vi "Setting.vi"() -> ()   [LabVIEW 2020]
uses:
  <userlib>/_MGI/1D Array/MGI Average/MGI Average (DBL[]).vi
  Libraries/S7/S7.lvlib
panel:
  in  "输出轴大量程标定":bool
  in  "停止":bool
  in  "输出轴小量程标定":bool
  in  "输入轴标定":bool
  out "标定曲线":cluster{dbl[], dbl[]}[](graph)
  # "配置标定"
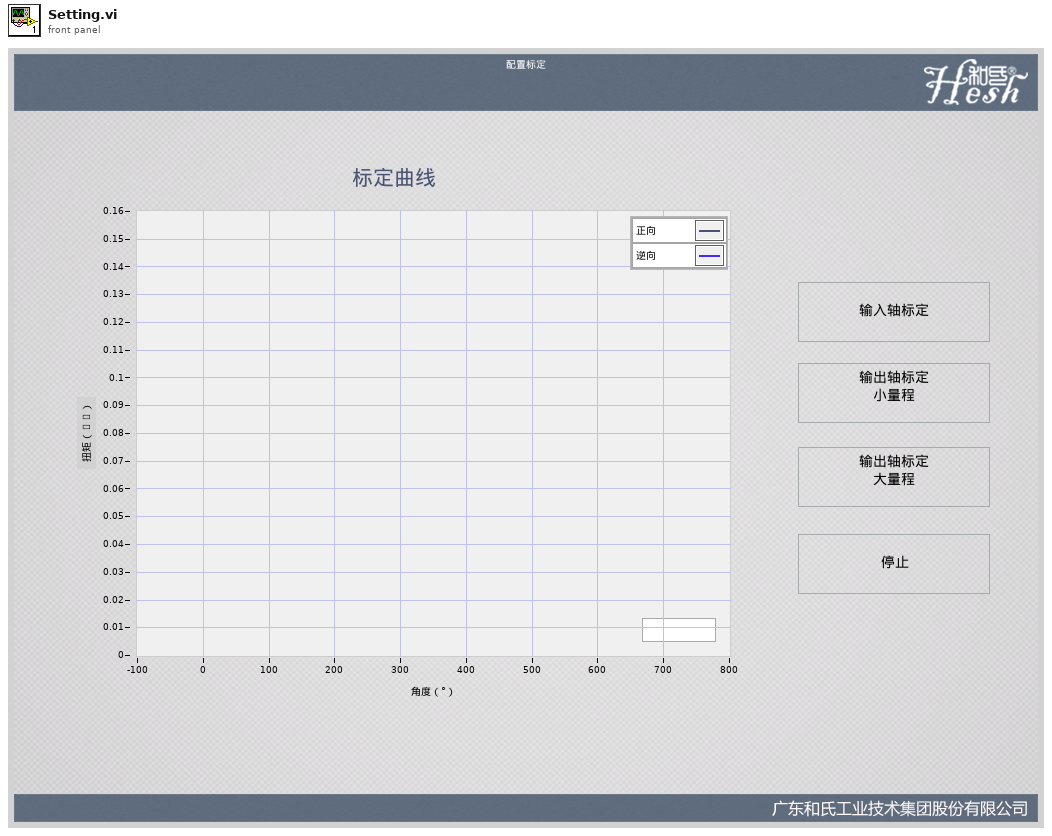
[diagram p1: front panel]
types:
  T1 = cluster{"输入旋转位移":sgl, "输入移载位移":sgl, "工装移载位移":sgl, "输入编码位移":sgl, "输入扭矩":sgl, "输出扭矩(小)":sgl, "输出扭矩(大)":sgl, "吸收电流":sgl, "Factorysensor":sgl, "输出轴旋转角度":sgl, "输出轴移栽位移":sgl, "Factorysensor2":sgl}
  T2 = cluster{"输入轴扭矩":dbl, "输出轴扭矩小量程":dbl, "输出轴扭矩大量程":dbl}
  T3 = typedef "S7.lvlib/Read_Data (Reply Payload)--cluster.ctl" = cluster{"读取成功":bool, "数据":u32[], "Read_Data_error":errorcluster}
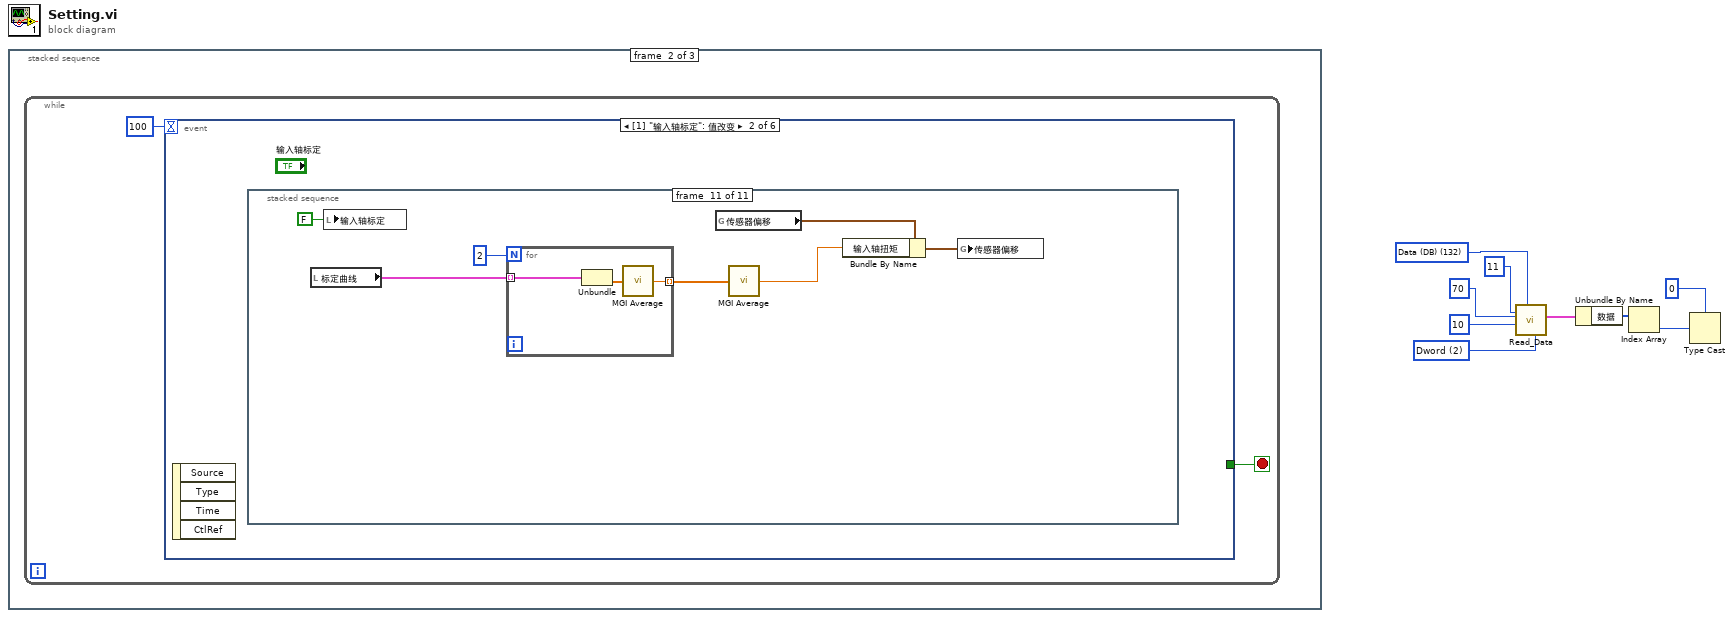
[diagram p0: block diagram]
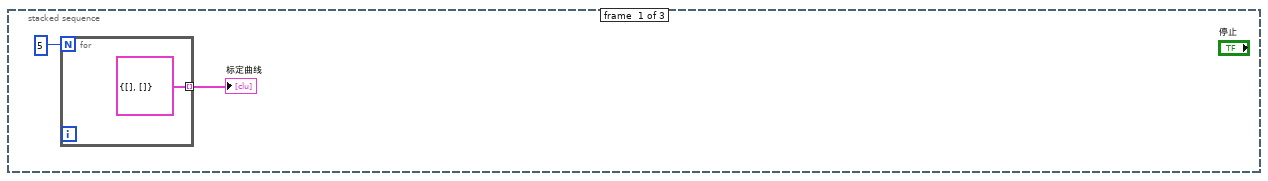
[diagram p2: hidden frame]
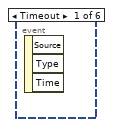
[diagram p3: hidden frame]
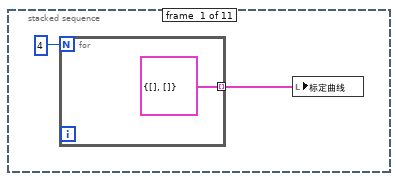
[diagram p4: hidden frame]
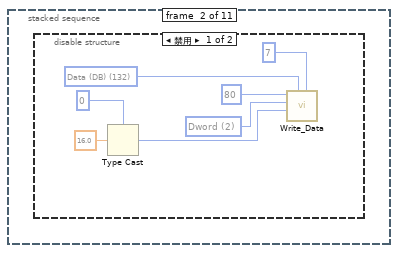
[diagram p5: hidden frame]
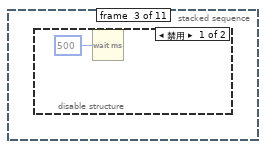
[diagram p7: hidden frame]
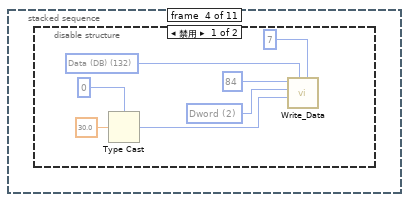
[diagram p9: hidden frame]
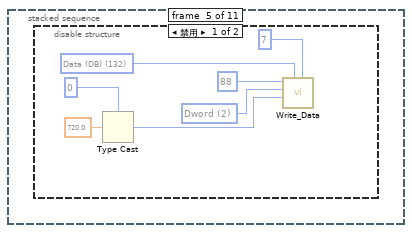
[diagram p11: hidden frame]
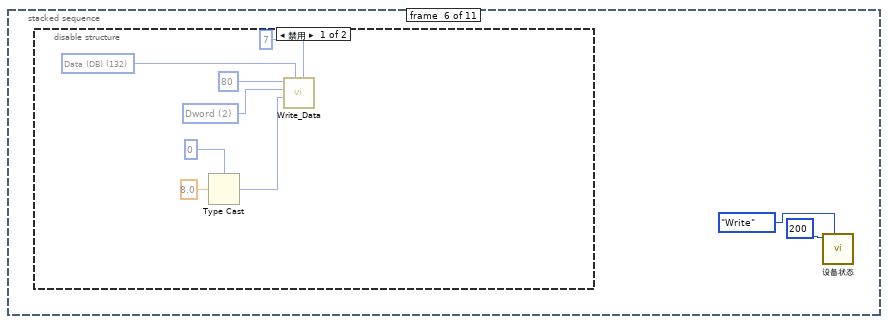
[diagram p13: hidden frame]
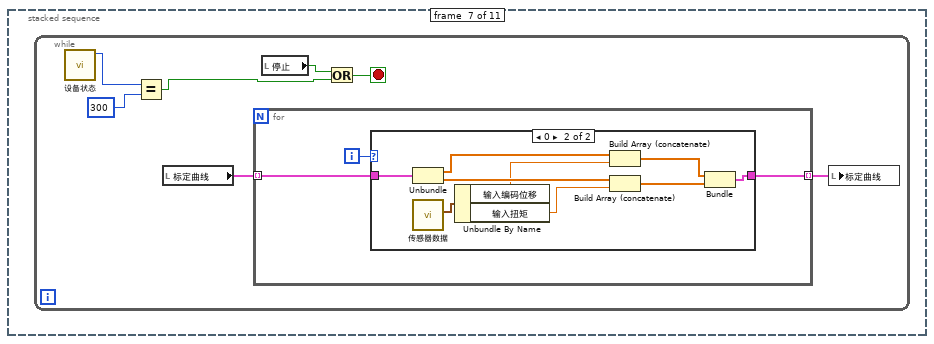
[diagram p15: hidden frame]
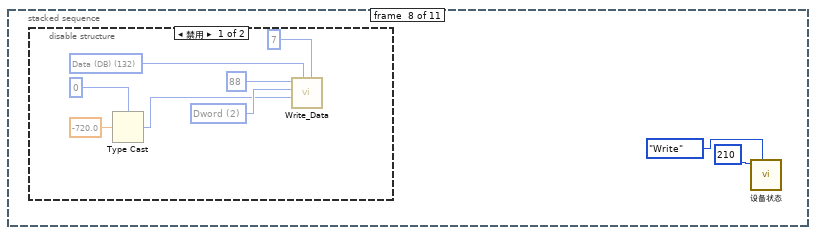
[diagram p17: hidden frame]
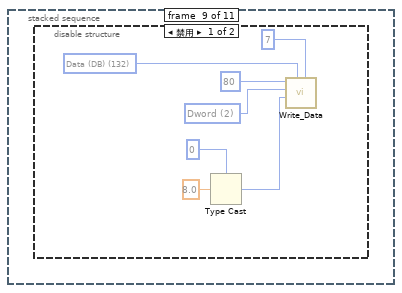
[diagram p19: hidden frame]
diagram:
  w6 = u16 2 items=["byte", "word", "Dword"] ("数据类型")
  w7 = u8 132 items=["I/O (P)"=128, "Input (I)"=129, "Output (Q)"=130, "Bit Memory (M)"=131, "Data (DB)"=132, "Instance Data (DI)"=133, "Local Data (L)"=134, "Predecessor Local Data (VL)"=135] ("寄存器类型")
  n1 = stacked-sequence {
    frame #0 {
      n2 = for {
        N: 5 -> [_]
        tunnel: [cluster{dbl[], dbl[]} {[], []}] -> w10 mode=indexing
      }
      "标定曲线" <- w10
    }
    frame #1 {
      n3 = while {
        stop <- w14 stop-if-true
        n4 = event shown="[1] \"输入轴标定\": 值改变" {
          selector: _ -> [_ _ _ _ _ _]
          dyn-events: _ -> [_ _ _ _ _ _]
          timeout: 100 -> [_ _ _ _ _ _]
          tunnel: [_ _ _ _ TRUE _] -> w14
          event Timeout {
            n5 = event-data() -> ()  [unwired: 1 in, 3 out]
          }
          event "输入轴标定": Value Change {
            n6 = event-data() -> ()  [unwired: 1 in, 4 out]
            n7 = stacked-sequence {
              frame #0 {
                n8 = for {
                  N: 4 -> [_]
                  tunnel: [cluster{dbl[], dbl[]} {[], []}] -> w16 mode=indexing
                }
                n9 = local write "标定曲线"(w16) -> ()
              }
              frame #1 {
                n10 = disable-structure shown="禁用" {
                  frame Disabled {
                    w22 = u16 2 items=["byte", "word", "Dword"] ("数据类型")
                    w24 = u8 132 items=["I/O (P)"=128, "Input (I)"=129, "Output (Q)"=130, "Bit Memory (M)"=131, "Data (DB)"=132, "Instance Data (DI)"=133, "Local Data (L)"=134, "Predecessor Local Data (VL)"=135] ("寄存器类型")
                    n11 = Type Cast(type=u32 0, x=sgl 16.0 ("输入轴旋转绝对位置")) -> (*(type *) &x=w20:u32)
                    n12 = call "Write_Data.vi"("DB #"=u16 7, "寄存器类型"=w24, "写入数据"=w20, "数据类型"=w22, "写入地址"=u32 80) -> ()  [unwired: 4 in, 3 out]
                  }
                  frame Enabled {
                  }
                }
              }
              frame #2 {
                n13 = disable-structure shown="禁用" {
                  frame Disabled {
                    n14 = Wait (ms)(milliseconds to wait=u32 500 ("等待时间（毫秒）")) -> ()  [unwired: 1 out]
                  }
                  frame Enabled {
                  }
                }
              }
              frame #3 {
                n15 = disable-structure shown="禁用" {
                  frame Disabled {
                    w30 = u16 2 items=["byte", "word", "Dword"] ("数据类型")
                    w32 = u8 132 items=["I/O (P)"=128, "Input (I)"=129, "Output (Q)"=130, "Bit Memory (M)"=131, "Data (DB)"=132, "Instance Data (DI)"=133, "Local Data (L)"=134, "Predecessor Local Data (VL)"=135] ("寄存器类型")
                    n16 = Type Cast(type=u32 0, x=sgl 30.0 ("输入轴旋转绝对位置")) -> (*(type *) &x=w28:u32)
                    n17 = call "Write_Data.vi"("DB #"=u16 7, "寄存器类型"=w32, "写入数据"=w28, "数据类型"=w30, "写入地址"=u32 84) -> ()  [unwired: 4 in, 3 out]
                  }
                  frame Enabled {
                  }
                }
              }
              frame #4 {
                n18 = disable-structure shown="禁用" {
                  frame Disabled {
                    w36 = u16 2 items=["byte", "word", "Dword"] ("数据类型")
                    w37 = u8 132 items=["I/O (P)"=128, "Input (I)"=129, "Output (Q)"=130, "Bit Memory (M)"=131, "Data (DB)"=132, "Instance Data (DI)"=133, "Local Data (L)"=134, "Predecessor Local Data (VL)"=135] ("寄存器类型")
                    n19 = Type Cast(type=u32 0, x=sgl 720.0 ("输入轴旋转绝对位置")) -> (*(type *) &x=w39:u32)
                    n20 = call "Write_Data.vi"("DB #"=u16 7, "寄存器类型"=w37, "写入数据"=w39, "数据类型"=w36, "写入地址"=u32 88) -> ()  [unwired: 4 in, 3 out]
                  }
                  frame Enabled {
                  }
                }
              }
              frame #5 {
                n21 = disable-structure shown="禁用" {
                  frame Disabled {
                    w45 = u16 2 items=["byte", "word", "Dword"] ("数据类型")
                    w46 = u8 132 items=["I/O (P)"=128, "Input (I)"=129, "Output (Q)"=130, "Bit Memory (M)"=131, "Data (DB)"=132, "Instance Data (DI)"=133, "Local Data (L)"=134, "Predecessor Local Data (VL)"=135] ("寄存器类型")
                    n22 = Type Cast(type=u32 0, x=sgl 8.0 ("输入轴旋转绝对位置")) -> (*(type *) &x=w48:u32)
                    n23 = call "Write_Data.vi"("DB #"=u16 7, "寄存器类型"=w46, "写入数据"=w48, "数据类型"=w45, "写入地址"=u32 80) -> ()  [unwired: 4 in, 3 out]
                  }
                  frame Enabled {
                  }
                }
                n24 = call "设备状态.vi"("枚举"=enum16{"Read", "Write"}."Write", "Status_Write"=i16 200 ("设备状态")) -> ()  [unwired: 9 in, 1 out]
              }
              frame #6 {
                n25 = while {
                  stop <- w54 stop-if-true
                  n26 = call "设备状态.vi"() -> ("Status_Read"=w49:i16)  [unwired: 11 in]
                  n27 = Equal?(x=w49, y=i16 300) -> (x = y?=w51:bool)
                  n28 = local read "标定曲线"() -> (w53:cluster{dbl[], dbl[]}[])
                  n29 = for {
                    tunnel: [w56] -> w52 mode=indexing
                    tunnel: w53 -> [w58] mode=indexing
                    i -> [w57]
                    n30 = case shown="0" w57 {
                      tunnel: [w59 w63] -> w56
                      tunnel: w58 -> [w59 w64]
                      frame Default {
                      }
                      frame 0 {
                        n31 = Unbundle(w64) -> (w68:dbl[], w67:dbl[])
                        n32 = call "传感器数据.vi"() -> ("PLCchuanganqishuju"=w60:T1)  [unwired: 10 in, 1 out]
                        n33 = Unbundle By Name(w60) -> ("输入编码位移"=w62:sgl, "输入扭矩"=w61:sgl)
                        n34 = Build Array (concatenate)(w68, w62) -> (w66:dbl[])
                        n35 = Build Array (concatenate)(w67, w61) -> (w65:dbl[])
                        n36 = Bundle(w66, w65) -> (w63:cluster{dbl[], dbl[]})  [unwired: 1 in]
                      }
                    }
                  }
                  n37 = local read "停止"() -> (w55:bool)
                  n38 = Or(x=w55, y=w51) -> (x .or. y?=w54:bool)
                  n39 = local write "标定曲线"(w52) -> ()
                }
              }
              frame #7 {
                n40 = disable-structure shown="禁用" {
                  frame Disabled {
                    w75 = u16 2 items=["byte", "word", "Dword"] ("数据类型")
                    w77 = u8 132 items=["I/O (P)"=128, "Input (I)"=129, "Output (Q)"=130, "Bit Memory (M)"=131, "Data (DB)"=132, "Instance Data (DI)"=133, "Local Data (L)"=134, "Predecessor Local Data (VL)"=135] ("寄存器类型")
                    n41 = Type Cast(type=u32 0, x=sgl -720.0 ("输入轴旋转绝对位置")) -> (*(type *) &x=w73:u32)
                    n42 = call "Write_Data.vi"("DB #"=u16 7, "寄存器类型"=w77, "写入数据"=w73, "数据类型"=w75, "写入地址"=u32 88) -> ()  [unwired: 4 in, 3 out]
                  }
                  frame Enabled {
                  }
                }
                n43 = call "设备状态.vi"("枚举"=enum16{"Read", "Write"}."Write", "Status_Write"=i16 210 ("设备状态")) -> ()  [unwired: 9 in, 1 out]
              }
              frame #8 {
                n44 = disable-structure shown="禁用" {
                  frame Disabled {
                    w82 = u16 2 items=["byte", "word", "Dword"] ("数据类型")
                    w84 = u8 132 items=["I/O (P)"=128, "Input (I)"=129, "Output (Q)"=130, "Bit Memory (M)"=131, "Data (DB)"=132, "Instance Data (DI)"=133, "Local Data (L)"=134, "Predecessor Local Data (VL)"=135] ("寄存器类型")
                    n45 = Type Cast(type=u32 0, x=sgl 8.0 ("输入轴旋转绝对位置")) -> (*(type *) &x=w80:u32)
                    n46 = call "Write_Data.vi"("DB #"=u16 7, "寄存器类型"=w84, "写入数据"=w80, "数据类型"=w82, "写入地址"=u32 80) -> ()  [unwired: 4 in, 3 out]
                  }
                  frame Enabled {
                  }
                }
              }
              frame #9 {
                n47 = while {
                  stop <- w91 stop-if-true
                  n48 = call "设备状态.vi"() -> ("Status_Read"=w86:i16)  [unwired: 11 in]
                  n49 = local read "标定曲线"() -> (w89:cluster{dbl[], dbl[]}[])
                  n50 = local read "停止"() -> (w90:bool)
                  n51 = Equal?(x=w86, y=i16 310) -> (x = y?=w85:bool)
                  n52 = Or(x=w85, y=w90) -> (x .or. y?=w91:bool)
                  n53 = for {
                    tunnel: [w92] -> w88 mode=indexing
                    tunnel: w89 -> [w94] mode=indexing
                    i -> [w93]
                    n54 = case shown="1" w93 {
                      tunnel: [w95 w99] -> w92
                      tunnel: w94 -> [w95 w100]
                      frame Default {
                      }
                      frame 1 {
                        n55 = Unbundle(w100) -> (w104:dbl[], w103:dbl[])
                        n56 = call "传感器数据.vi"() -> ("PLCchuanganqishuju"=w96:T1)  [unwired: 10 in, 1 out]
                        n57 = Unbundle By Name(w96) -> ("输入编码位移"=w97:sgl, "输入扭矩"=w98:sgl)
                        n58 = Build Array (concatenate)(w104, w97) -> (w102:dbl[])
                        n59 = Build Array (concatenate)(w103, w98) -> (w101:dbl[])
                        n60 = Bundle(w102, w101) -> (w99:cluster{dbl[], dbl[]})  [unwired: 1 in]
                      }
                    }
                  }
                  n61 = local write "标定曲线"(w88) -> ()
                }
              }
              frame #10 {
                n62 = local read "标定曲线"() -> (w106:cluster{dbl[], dbl[]}[])
                n63 = local write "输入轴标定"(FALSE ("输入轴标定")) -> ()
                n64 = for {
                  N: 2 -> [_]
                  tunnel: w106 -> [w114] mode=indexing
                  tunnel: [w112] -> w107 mode=indexing
                  n65 = Unbundle(w114) -> (w113:dbl[])  [unwired: 1 out]
                  n66 = call-poly <userlib>:"MGI Average.vi"("Double[]"=w113) -> ("Average"=w112:dbl)  [unwired: 1 in]
                }
                n67 = global read "传感器偏移.vi" "传感器偏移"() -> (w109:T2)
                n68 = call-poly <userlib>:"MGI Average.vi"("Double[]"=w107) -> ("Average"=w105:dbl)  [unwired: 1 in]
                n69 = Bundle By Name(cluster=w109, "输入轴扭矩"=w105) -> (w110:T2)
                n70 = global write "传感器偏移.vi" "传感器偏移"(w110) -> ()
              }
            }
          }
          event "输出轴小量程标定": Value Change {
            n71 = event-data() -> ()  [unwired: 1 in, 4 out]
            n72 = stacked-sequence {
              frame #0 {
                n73 = disable-structure shown="禁用" {
                  frame Disabled {
                    n74 = call "SetActualPosition.vi"() -> ()  [unwired: 11 in, 1 out]
                  }
                  frame Enabled {
                  }
                }
              }
              frame #1 {
                n75 = for {
                  N: 4 -> [_]
                  tunnel: [cluster{dbl[], dbl[]} {[], []}] -> w116 mode=indexing
                }
                n76 = local write "标定曲线"(w116) -> ()
              }
              frame #2 {
                n77 = disable-structure shown="禁用" {
                  frame Disabled {
                    n78 = call-poly "模式选择.vi"("Max Torque"=100.0, "Velocity"=30.0) -> ()  [unwired: 9 in, 1 out]
                  }
                  frame Enabled {
                  }
                }
                n79 = call "设备状态.vi"("枚举"=enum16{"Read", "Write"}."Write", "Status_Write"=i16 201 ("设备状态")) -> ()  [unwired: 9 in, 1 out]
              }
              frame #3 {
                n80 = while {
                  stop <- w126 stop-if-true
                  n81 = call "设备状态.vi"() -> ("Status_Read"=w123:i16)  [unwired: 11 in]
                  n82 = call "传感器数据.vi"() -> ("PLCchuanganqishuju"=w122:T1)  [unwired: 10 in, 1 out]
                  n83 = Unbundle By Name(w122) -> ("输出扭矩(小)"=w129:sgl, "输出轴旋转角度"=w128:sgl)
                  n84 = Equal?(x=w123, y=i16 301) -> (x = y?=w125:bool)
                  n85 = local read "停止"() -> (w124:bool)
                  n86 = control-ref of="标定曲线"() -> (w130:refnum<vi>)
                  n87 = Or(x=w124, y=w125) -> (x .or. y?=w126:bool)
                  n88 = call "曲线采集.vi"("曲线引用"=w130, "曲线索引"=0, "X"=w128, "Y"=w129) -> ()  [unwired: 10 in, 2 out]
                }
              }
              frame #4 {
                n89 = disable-structure shown="禁用" {
                  frame Disabled {
                    n90 = call-poly "模式选择.vi"("Max Torque"=100.0, "Velocity"=-30.0) -> ()  [unwired: 9 in, 1 out]
                  }
                  frame Enabled {
                  }
                }
                n91 = call "设备状态.vi"("枚举"=enum16{"Read", "Write"}."Write", "Status_Write"=i16 211 ("设备状态")) -> ()  [unwired: 9 in, 1 out]
              }
              frame #5 {
                n92 = while {
                  stop <- w138 stop-if-true
                  n93 = call "传感器数据.vi"() -> ("PLCchuanganqishuju"=w136:T1)  [unwired: 10 in, 1 out]
                  n94 = Unbundle By Name(w136) -> ("输出扭矩(小)"=w143:sgl, "输出轴旋转角度"=w142:sgl)
                  n95 = control-ref of="标定曲线"() -> (w144:refnum<vi>)
                  n96 = call "曲线采集.vi"("曲线引用"=w144, "曲线索引"=1, "X"=w142, "Y"=w143) -> ()  [unwired: 10 in, 2 out]
                  n97 = call "设备状态.vi"() -> ("Status_Read"=w140:i16)  [unwired: 11 in]
                  n98 = local read "停止"() -> (w139:bool)
                  n99 = Equal?(x=w140, y=i16 311) -> (x = y?=w137:bool)
                  n100 = Or(x=w139, y=w137) -> (x .or. y?=w138:bool)
                }
              }
              frame #6 {
                n101 = local write "输出轴小量程标定"(FALSE ("输入轴标定")) -> ()
                n102 = disable-structure shown="禁用" {
                  frame Disabled {
                    n103 = call-poly "模式选择.vi"() -> ()  [unwired: 11 in, 1 out]
                  }
                  frame Enabled {
                  }
                }
              }
              frame #7 {
                n104 = local read "标定曲线"() -> (w147:cluster{dbl[], dbl[]}[])
                n105 = for {
                  N: 2 -> [_]
                  tunnel: w147 -> [w155] mode=indexing
                  tunnel: [w153] -> w148 mode=indexing
                  n106 = Unbundle(w155) -> (w154:dbl[])  [unwired: 1 out]
                  n107 = call-poly <userlib>:"MGI Average.vi"("Double[]"=w154) -> ("Average"=w153:dbl)  [unwired: 1 in]
                }
                n108 = global read "传感器偏移.vi" "传感器偏移"() -> (w150:T2)
                n109 = call-poly <userlib>:"MGI Average.vi"("Double[]"=w148) -> ("Average"=w152:dbl)  [unwired: 1 in]
                n110 = Bundle By Name(cluster=w150, "输出轴扭矩小量程"=w152) -> (w151:T2)
                n111 = global write "传感器偏移.vi" "传感器偏移"(w151) -> ()
              }
            }
          }
          event "输出轴大量程标定": Value Change {
            n112 = event-data() -> ()  [unwired: 1 in, 4 out]
            n113 = stacked-sequence {
              frame #0 {
                n114 = disable-structure shown="禁用" {
                  frame Disabled {
                    n115 = call "SetActualPosition.vi"() -> ()  [unwired: 11 in, 1 out]
                  }
                  frame Enabled {
                  }
                }
              }
              frame #1 {
                n116 = for {
                  N: 4 -> [_]
                  tunnel: [cluster{dbl[], dbl[]} {[], []}] -> w157 mode=indexing
                }
                n117 = local write "标定曲线"(w157) -> ()
              }
              frame #2 {
                n118 = disable-structure shown="禁用" {
                  frame Disabled {
                    n119 = call-poly "模式选择.vi"("Max Torque"=100.0, "Velocity"=30.0) -> ()  [unwired: 9 in, 1 out]
                  }
                  frame Enabled {
                  }
                }
                n120 = call "设备状态.vi"("枚举"=enum16{"Read", "Write"}."Write", "Status_Write"=i16 202 ("设备状态")) -> ()  [unwired: 9 in, 1 out]
              }
              frame #3 {
                n121 = while {
                  stop <- w168 stop-if-true
                  n122 = call "传感器数据.vi"() -> ("PLCchuanganqishuju"=w163:T1)  [unwired: 10 in, 1 out]
                  n123 = call "设备状态.vi"() -> ("Status_Read"=w164:i16)  [unwired: 11 in]
                  n124 = Equal?(x=w164, y=i16 302) -> (x = y?=w165:bool)
                  n125 = Unbundle By Name(w163) -> ("输出扭矩(大)"=w170:sgl, "输出轴旋转角度"=w169:sgl)
                  n126 = local read "停止"() -> (w167:bool)
                  n127 = control-ref of="标定曲线"() -> (w172:refnum<vi>)
                  n128 = Or(x=w167, y=w165) -> (x .or. y?=w168:bool)
                  n129 = call "曲线采集.vi"("曲线引用"=w172, "曲线索引"=0, "X"=w169, "Y"=w170) -> ()  [unwired: 10 in, 2 out]
                }
              }
              frame #4 {
                n130 = disable-structure shown="禁用" {
                  frame Disabled {
                    n131 = call-poly "模式选择.vi"("Max Torque"=100.0, "Velocity"=-30.0) -> ()  [unwired: 9 in, 1 out]
                  }
                  frame Enabled {
                  }
                }
                n132 = call "设备状态.vi"("枚举"=enum16{"Read", "Write"}."Write", "Status_Write"=i16 212 ("设备状态")) -> ()  [unwired: 9 in, 1 out]
              }
              frame #5 {
                n133 = while {
                  stop <- w178 stop-if-true
                  n134 = call "传感器数据.vi"() -> ("PLCchuanganqishuju"=w177:T1)  [unwired: 10 in, 1 out]
                  n135 = Unbundle By Name(w177) -> ("输出扭矩(大)"=w184:sgl, "输出轴旋转角度"=w183:sgl)
                  n136 = control-ref of="标定曲线"() -> (w185:refnum<vi>)
                  n137 = call "曲线采集.vi"("曲线引用"=w185, "曲线索引"=1, "X"=w183, "Y"=w184) -> ()  [unwired: 10 in, 2 out]
                  n138 = call "设备状态.vi"() -> ("Status_Read"=w182:i16)  [unwired: 11 in]
                  n139 = local read "停止"() -> (w180:bool)
                  n140 = Equal?(x=w182, y=i16 312) -> (x = y?=w181:bool)
                  n141 = Or(x=w180, y=w181) -> (x .or. y?=w178:bool)
                }
              }
              frame #6 {
                n142 = local write "输出轴大量程标定"(FALSE ("输入轴标定")) -> ()
                n143 = disable-structure shown="禁用" {
                  frame Disabled {
                    n144 = call-poly "模式选择.vi"() -> ()  [unwired: 11 in, 1 out]
                  }
                  frame Enabled {
                  }
                }
              }
              frame #7 {
                n145 = local read "标定曲线"() -> (w188:cluster{dbl[], dbl[]}[])
                n146 = for {
                  N: 2 -> [_]
                  tunnel: w188 -> [w196] mode=indexing
                  tunnel: [w194] -> w189 mode=indexing
                  n147 = Unbundle(w196) -> (w195:dbl[])  [unwired: 1 out]
                  n148 = call-poly <userlib>:"MGI Average.vi"("Double[]"=w195) -> ("Average"=w194:dbl)  [unwired: 1 in]
                }
                n149 = global read "传感器偏移.vi" "传感器偏移"() -> (w191:T2)
                n150 = call-poly <userlib>:"MGI Average.vi"("Double[]"=w189) -> ("Average"=w193:dbl)  [unwired: 1 in]
                n151 = Bundle By Name(cluster=w191, "输出轴扭矩大量程"=w193) -> (w192:T2)
                n152 = global write "传感器偏移.vi" "传感器偏移"(w192) -> ()
              }
            }
          }
          event Panel Close {
            n153 = event-data() -> ()  [unwired: 1 in, 4 out]
          }
          event "停止": Value Change {
            w198 = FALSE ("输出轴大量程标定")
            n154 = event-data() -> ()  [unwired: 1 in, 4 out]
            n155 = local write "输出轴小量程标定"(w198) -> ()
            n156 = local write "输出轴大量程标定"(w198) -> ()
            n157 = local write "输入轴标定"(w198) -> ()
          }
        }
      }
    }
    frame #2 {
      n158 = global read "传感器偏移.vi" "传感器偏移"() -> (w200:T2)
      n159 = call "Demarcate.vi"("Mode"=enum16{"Read", "Write"}."Write", "Sensor IN"=w200) -> ()  [unwired: 8 in, 2 out]
    }
  }
  n160 = call "Read_Data.vi"("数据类型"=w6, "读取长度"=u16 11, "寄存器类型"=w7, "起始地址"=u32 10, "DB #"=u16 70) -> ("Reply Payload"=w1:T3)  [unwired: 4 in, 2 out]
  n161 = Unbundle By Name(w1) -> ("数据"=w4:u32[])
  n162 = Index Array(array=w4) -> (element=w2:u32)  [unwired: 1 in]
  n163 = Type Cast(type=u32 0, x=w2) -> ()  [unwired: 1 out]
